vi "ICE450UltraMonitor.vi"(10 "delay before read (ms)":u32=500, 11 "VISA resource name":refnum<visa-resource-name>="COM7") -> ()   [LabVIEW 2016]
panel:
  in  "error in (no error)":errorcluster
  in  "CLOSE":bool
  out "Coolant level":string="ok\r\nLEV  OK        "
  out "Coolant level label":string="coolant level:"
  out "Pump flowrate":string="0 lpm\r\nFLOW "
  out "Pump flowrate label":string="pump flowrate:"
  out "Pump mode":string="normal"
  out "Pump mode label":string="pump mode:"
  out "Pump status":string="ON"
  out "Pump status label":string="pump status:"
  out "Pump label":string="pump"
  out "µs":string="uS"
  out "Q-switch delay label":string="Q-switch delay:"
  out "Q-switch delay":string="0"
  in  "Temperatures":string="temperatures"
  out "Flashlamp and Q-Switch":string="flashlamp - q-switch"
  out "FL voltage label":string="flashlamp voltage:\n"
  out "FL voltage":string="0 V"
  out "FL energy label":string="flashlamp energy:"
  out "FL energy":string="0.0 J"
  out "FL current":string="flashlamp total shots:"
  out "FL total":string="000000000"
  out "FL count total":string="flashlamp current shots:"
  out "FL current":string="000000000"
  in  "Degree symbol 3":string
  in  "Degree Celsius 3":string
  in  "Charger/Simmer":string="charger/simmer"
  out "Charger/simmer":dbl format="%.1g"
  in  "Degree symbol 2":string
  in  "Degree Celsius 2":string
  in  "Harmonic Generator":string="harmonic generator"
  out "Harmonic Generator":dbl format="%.1g"
  in  "Degree symbol":string
  in  "Degree Celsius":string
  in  "Cooling System":string="Cooling\ngroup"
  out "Cooling group":dbl format="%.1g"
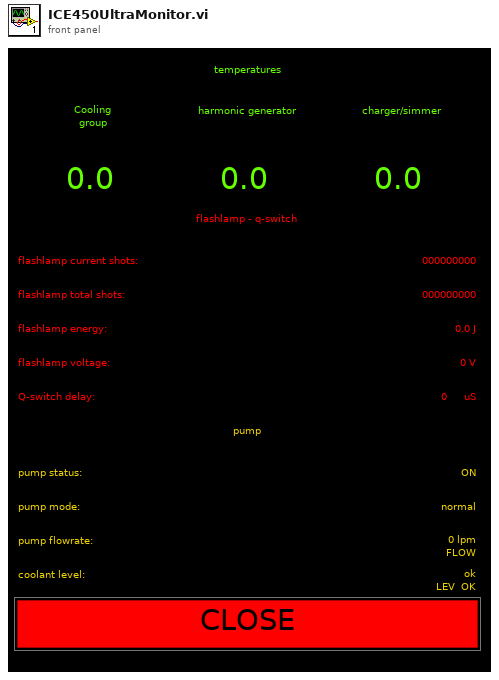
[diagram p1: front panel]
types:
  T1 = enum16{"Initialize", "FLCount", "FLCountTotal", "FLEnergy", "FLVoltage", "QSDelay", "PumpCheck", "PumpMode", "Flowrate", "CoolantLevel", "Temp", "Close"}
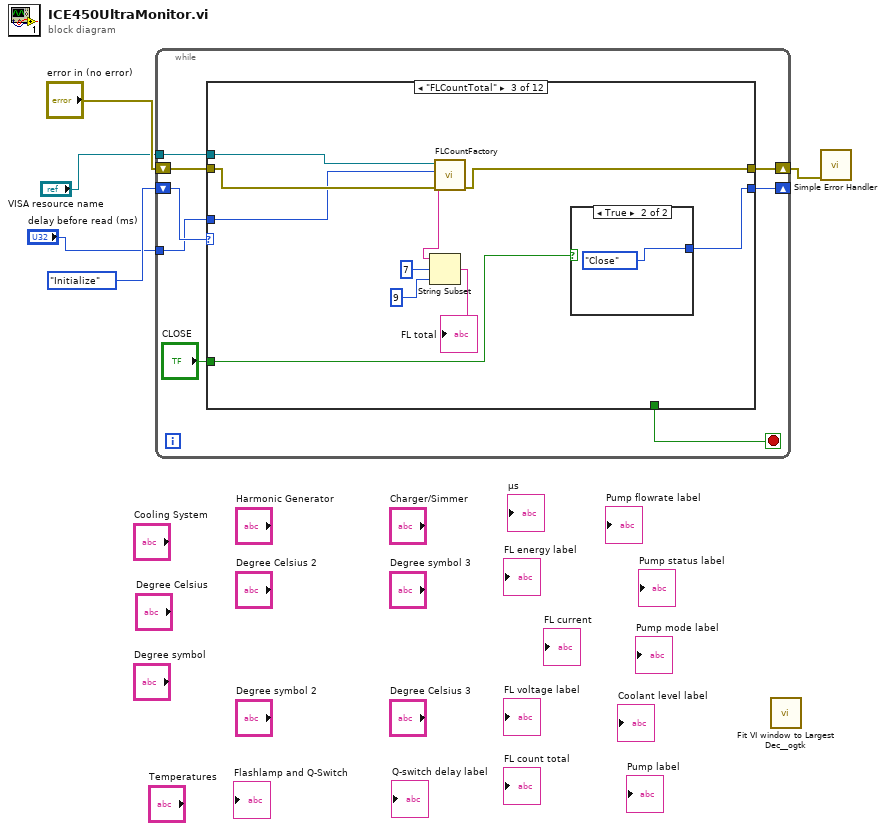
[diagram p0: block diagram]
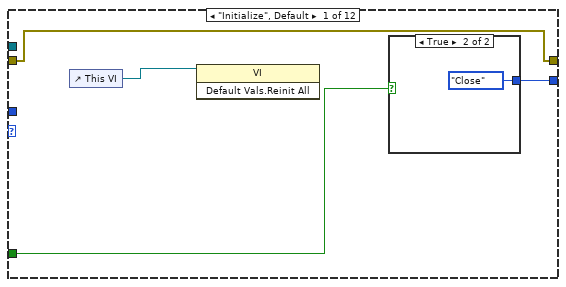
[diagram p2: hidden frame]
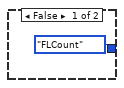
[diagram p3: hidden frame]
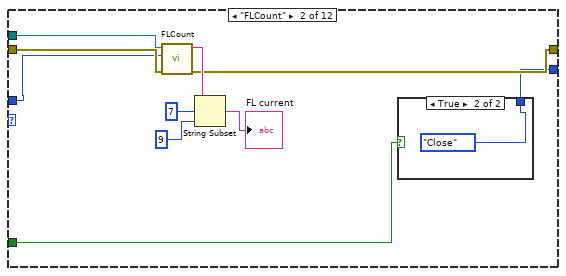
[diagram p4: hidden frame]
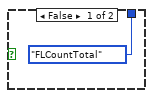
[diagram p5: hidden frame]
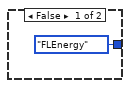
[diagram p6: hidden frame]
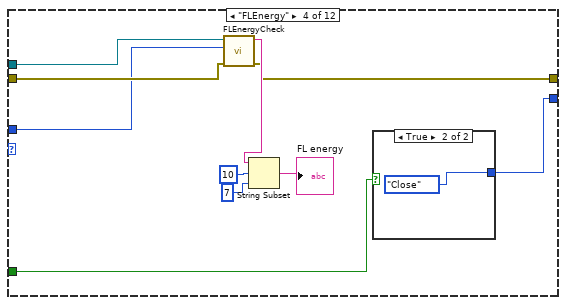
[diagram p7: hidden frame]
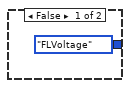
[diagram p8: hidden frame]
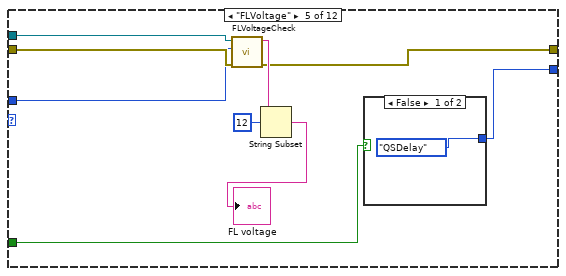
[diagram p9: hidden frame]
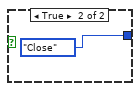
[diagram p10: hidden frame]
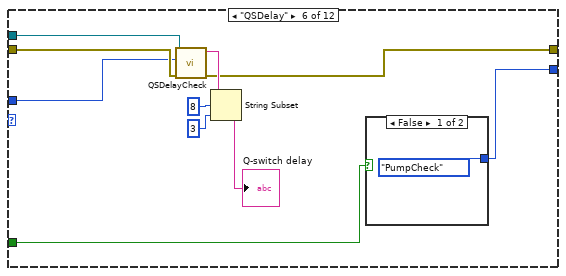
[diagram p11: hidden frame]
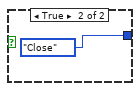
[diagram p12: hidden frame]
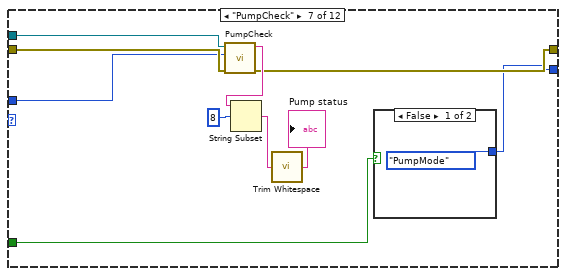
[diagram p13: hidden frame]
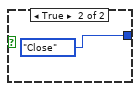
[diagram p14: hidden frame]
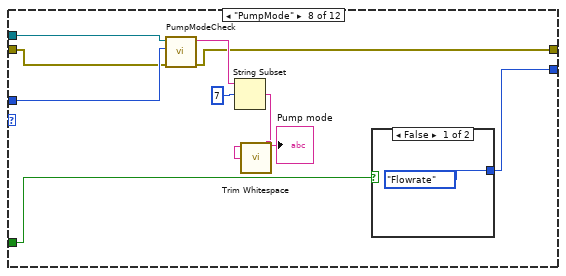
[diagram p15: hidden frame]
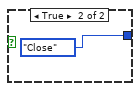
[diagram p16: hidden frame]
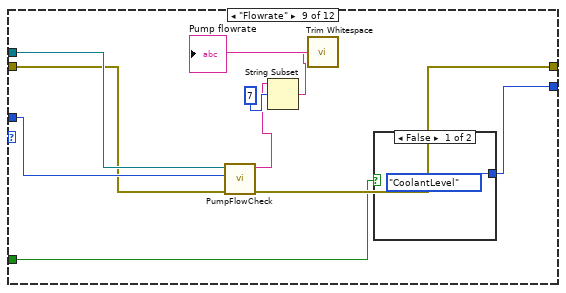
[diagram p17: hidden frame]
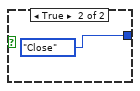
[diagram p18: hidden frame]
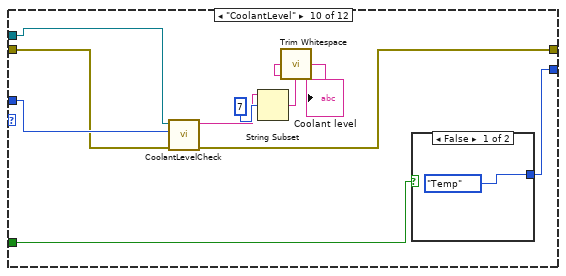
[diagram p19: hidden frame]
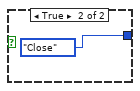
[diagram p20: hidden frame]
diagram:
  n1 = while {
    shift-right: [w12] -> _
    shift-left: T1."Initialize" -> [w13]
    shift-right: [w10] -> w4
    shift-left: "error in (no error)" -> [w11]
    tunnel: "VISA resource name" -> [w8]
    tunnel: "delay before read (ms)" -> [w7]
    stop <- w6 stop-if-true
    n2 = case shown="\"FLCountTotal\"" w13 {
      tunnel: [w16 w23 w32 w45 w58 w68 w80 w91 w104 w115 w127 T1."Close"] -> w12
      tunnel: w11 -> [w14 w25 w37 w49 w62 w72 w84 w94 w106 w118 w131 w153]
      tunnel: [w14 w24 w36 w46 w59 w69 w81 w93 w105 w117 w129 w153] -> w10
      tunnel: "CLOSE" -> [w15 w22 w33 w44 w57 w67 w79 w92 w103 w116 w128 _]
      tunnel: w8 -> [_ w21 w35 w48 w61 w71 w83 w96 w108 w120 w132 _]
      tunnel: w7 -> [_ w20 w34 w47 w60 w70 w82 w95 w107 w119 w130 _]
      tunnel: [_ _ _ _ _ _ _ _ _ _ _ TRUE] -> w6
      frame "Initialize", Default {
        n3 = control-ref of="This VI"() -> (w17:refnum<vi>)
        n4 = invoke class="VI" method="Default Vals.Reinit All"(reference=w17) -> ()  [unwired: 2 in, 3 out]
        n5 = case shown="True" w15 {
          tunnel: [T1."FLCount" T1."Close"] -> w16
          frame False {
          }
          frame True {
          }
        }
      }
      frame "FLCount" {
        n6 = call "FLCount.vi"("Error In"=w25, "delay before read (ms)"=w20, "VISA resource name"=w21) -> ("Error Out"=w24:errorcluster, "read buffer"=w27:string)  [unwired: 5 in, 2 out]
        n7 = String Subset(string=w27, offset (0)=7, length (rest)=9 ("length (rest)")) -> (substring=→"FL current":string)
        n8 = case shown="True" w22 {
          tunnel: [T1."FLCountTotal" T1."Close"] -> w23
          frame False {
          }
          frame True {
          }
        }
      }
      frame "FLCountTotal" {
        n9 = call "FLCountFactory.vi"("Error In"=w37, "delay before read (ms)"=w34, "VISA resource name"=w35) -> ("Error Out"=w36:errorcluster, "read buffer"=w40:string)  [unwired: 5 in, 2 out]
        n10 = String Subset(string=w40, offset (0)=7, length (rest)=9 ("length (rest)")) -> (substring=→"FL total":string)
        n11 = case shown="True" w33 {
          tunnel: [T1."FLEnergy" T1."Close"] -> w32
          frame False {
          }
          frame True {
          }
        }
      }
      frame "FLEnergy" {
        n12 = call "FLEnergyCheck.vi"("Error In"=w49, "delay before read (ms)"=w47, "VISA resource name"=w48) -> ("Error Out"=w46:errorcluster, "read buffer"=w51:string)  [unwired: 5 in, 2 out]
        n13 = String Subset(string=w51, offset (0)=10, length (rest)=7 ("length (rest)")) -> (substring=→"FL energy":string)
        n14 = case shown="True" w44 {
          tunnel: [T1."FLVoltage" T1."Close"] -> w45
          frame False {
          }
          frame True {
          }
        }
      }
      frame "FLVoltage" {
        n15 = call "FLVoltageCheck.vi"("Error In"=w62, "delay before read (ms)"=w60, "VISA resource name"=w61) -> ("Error Out"=w59:errorcluster, "read buffer"=w64:string)  [unwired: 5 in, 2 out]
        n16 = String Subset(string=w64, offset (0)=12) -> (substring=→"FL voltage":string)  [unwired: 1 in]
        n17 = case shown="False" w57 {
          tunnel: [T1."QSDelay" T1."Close"] -> w58
          frame False {
          }
          frame True {
          }
        }
      }
      frame "QSDelay" {
        n18 = call "QSDelayCheck.vi"("Error In"=w72, "delay before read (ms)"=w70, "VISA resource name"=w71) -> ("Error Out"=w69:errorcluster, "read buffer"=w75:string)  [unwired: 5 in, 2 out]
        n19 = String Subset(string=w75, offset (0)=8, length (rest)=3 ("length (rest)")) -> (substring=→"Q-switch delay":string)
        n20 = case shown="False" w67 {
          tunnel: [T1."PumpCheck" T1."Close"] -> w68
          frame False {
          }
          frame True {
          }
        }
      }
      frame "PumpCheck" {
        n21 = call "PumpCheck.vi"("Error In"=w84, "delay before read (ms)"=w82, "VISA resource name"=w83) -> ("Error Out"=w81:errorcluster, "read buffer"=w86:string)  [unwired: 5 in, 2 out]
        n22 = String Subset(string=w86, offset (0)=8) -> (substring=w87:string)  [unwired: 1 in]
        n23 = call <vilib>:"Trim Whitespace.vi"("string"=w87) -> ("trimmed string"=→"Pump status":string)  [unwired: 1 in]
        n24 = case shown="False" w79 {
          tunnel: [T1."PumpMode" T1."Close"] -> w80
          frame False {
          }
          frame True {
          }
        }
      }
      frame "PumpMode" {
        n25 = call "PumpModeCheck.vi"("Error In"=w94, "delay before read (ms)"=w95, "VISA resource name"=w96) -> ("Error Out"=w93:errorcluster, "read buffer"=w98:string)  [unwired: 5 in, 2 out]
        n26 = String Subset(string=w98, offset (0)=7) -> (substring=w99:string)  [unwired: 1 in]
        n27 = call <vilib>:"Trim Whitespace.vi"("string"=w99) -> ("trimmed string"=→"Pump mode":string)  [unwired: 1 in]
        n28 = case shown="False" w92 {
          tunnel: [T1."Flowrate" T1."Close"] -> w91
          frame False {
          }
          frame True {
          }
        }
      }
      frame "Flowrate" {
        n29 = call "PumpFlowCheck.vi"("Error In"=w106, "delay before read (ms)"=w107, "VISA resource name"=w108) -> ("Error Out"=w105:errorcluster, "read buffer"=w109:string)  [unwired: 5 in, 2 out]
        n30 = String Subset(string=w109, offset (0)=7) -> (substring=w111:string)  [unwired: 1 in]
        n31 = call <vilib>:"Trim Whitespace.vi"("string"=w111) -> ("trimmed string"=→"Pump flowrate":string)  [unwired: 1 in]
        n32 = case shown="False" w103 {
          tunnel: [T1."CoolantLevel" T1."Close"] -> w104
          frame False {
          }
          frame True {
          }
        }
      }
      frame "CoolantLevel" {
        n33 = call "CoolantLevelCheck.vi"("Error In"=w118, "delay before read (ms)"=w119, "VISA resource name"=w120) -> ("Error Out"=w117:errorcluster, "read buffer"=w121:string)  [unwired: 5 in, 2 out]
        n34 = String Subset(string=w121, offset (0)=7) -> (substring=w123:string)  [unwired: 1 in]
        n35 = call <vilib>:"Trim Whitespace.vi"("string"=w123) -> ("trimmed string"=→"Coolant level":string)  [unwired: 1 in]
        n36 = case shown="False" w116 {
          tunnel: [T1."Temp" T1."Close"] -> w115
          frame False {
          }
          frame True {
          }
        }
      }
      frame "Temp" {
        w136 = 10 ("y")
        n37 = call "TempStatus.vi"("Error In"=w131, "delay before read (ms)"=w130, "VISA resource name"=w132) -> ("Error Out"=w129:errorcluster, "read buffer"=w149:string)  [unwired: 5 in, 2 out]
        n38 = String Subset(string=w149, offset (0)=9, length (rest)=3 ("length (rest)")) -> (substring=w140:string)
        n39 = String Subset(string=w149, offset (0)=5, length (rest)=3 ("length (rest)")) -> (substring=w141:string)
        n40 = String Subset(string=w149, offset (0)=13, length (rest)=3 ("length (rest)")) -> (substring=w142:string)
        n41 = Decimal String To Number(string=w140) -> (number=w137:i32)  [unwired: 2 in, 1 out]
        n42 = Decimal String To Number(string=w141) -> (number=w139:i32)  [unwired: 2 in, 1 out]
        n43 = Divide(x=w137, y=w136) -> (x/y=→"Harmonic Generator":dbl)
        n44 = Divide(x=w139, y=w136) -> (x/y=→"Cooling group":dbl)
        n45 = Decimal String To Number(string=w142) -> (number=w138:i32)  [unwired: 2 in, 1 out]
        n46 = Divide(x=w138, y=w136) -> (x/y=→"Charger/simmer":dbl)
        n47 = case shown="False" w128 {
          tunnel: [T1."FLCount" T1."Close"] -> w127
          frame False {
          }
          frame True {
          }
        }
      }
      frame "Close" {
      }
    }
  }
  n48 = call <userlib>:"Fit VI window to Largest Dec__ogtk.vi"() -> ()  [unwired: 6 in, 2 out]
  n49 = call <vilib>:"Simple Error Handler.vi"("error in (no error)"=w4) -> ()  [unwired: 4 in, 5 out]
